vi "ABR3-Channel Assignments.vi"(0 "Stimulus":T5={"Ear"=enum."Left", "Waveform"=enum."TONE PIP", "Frequency (kHz)"="", "Rep rate (/sec)"=30.0, "Alternate Polarity"=FALSE, "WavFiles"="", "Level (dB SPL)"=30.0, "WavFolder"=path "", "Chirp"={"Type"=enum."AN latency-corrected", "Duration (ms)"=0.0, "Fmin (kHz)"=0.0, "Fmax (kHz)"=0.0, "precompensate"=FALSE}, "Noise"={"Seed"=0, "InvFilt"=FALSE, "AWeight"=FALSE, "afile"=path "", "Filter"={"Type"=enum."Lowpass", "CF (kHz)"=0.0, "BW (kHz)"=0.0, "Cascade"=FALSE, "Quadrature"=FALSE, "Scale Factor"=0.0, "Stages"=[], "Class"=enum."Elliptic", "Order"=0, "BWUnits"=enum."Linear"}}}, 1 "Masker":T2, 11 "error in (no error)":errorcluster) -> (15 "error out":errorcluster)   [LabVIEW 2020]
uses:
  TypeDefs/ABR3-Stimulus.ctl
  Utility VIs/Type Defs/Left-Right ring.ctl
  TypeDefs/ABR-Waveform Enum.ctl
  Signal Synthesis VIs/Controls/Advanced Filter XCtl/Advanced Filter XCtl.xctl
  TypeDefs/ABR3-Masker Spec.ctl
  Signal Synthesis VIs/Controls/Level XCtl/Level XCtl.xctl
  Utility VIs/Type Defs/Speaker ring.ctl
panel:
  out "Masker channels":T1[](array[typedef])
  out "Unused secondary channels":T1[](array[typedef])
  out "Signal channels":T1[](array[typedef])
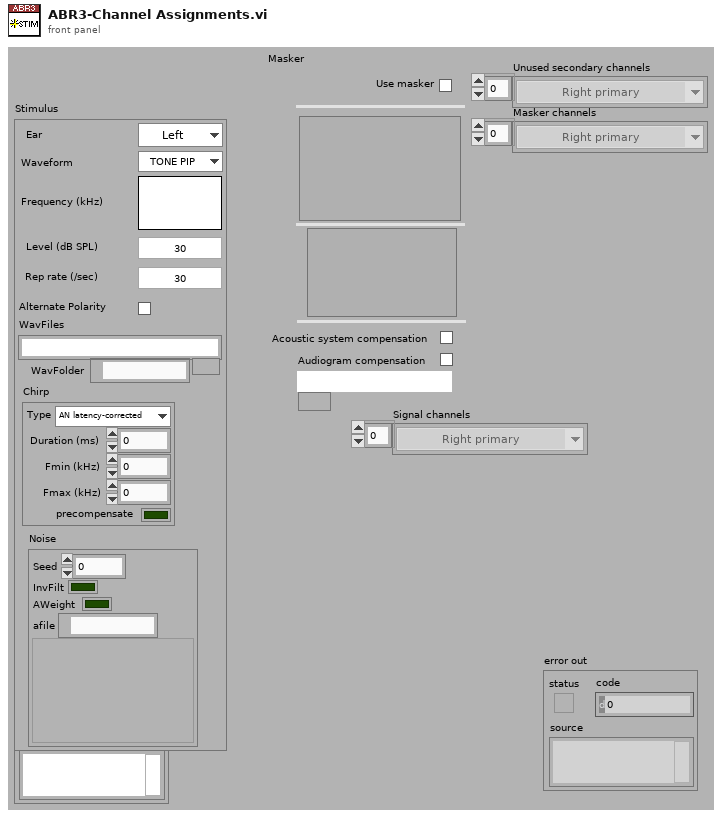
[diagram p1: front panel]
types:
  T1 = typedef "Speaker ring.ctl" = enum16{"Right primary", "Right secondary", "Left primary", "Left secondary"}
  T2 = typedef "ABR3-Masker Spec.ctl" = cluster{"Filter":cluster{"Type":enum16{"Lowpass", "Highpass", "Bandpass", "Bandstop", "OFF"}, "CF (kHz)":dbl, "BW (kHz)":dbl, "Cascade":bool, "Quadrature":bool, "Scale Factor":dbl, "Stages":cluster{"IIR Filter":cluster{"filter structure":enum32{"IIR 2nd Order", "IIR 4th Order"}, "Reverse Coefficients":dbl[], "Forward Coefficients":dbl[]}, "State":dbl[]}[], "Class":enum16{"Elliptic", "Butterworth"}, "Order":i32, "BWUnits":T3}, "Use masker":bool, "Level":cluster{"Level":dbl, "Units":T4, "Max":dbl, "Multiplier":dbl, "Cal File":path, "Cal":cluster{"Freq (Hz)":dbl[], "Mag (dB SPL)":dbl[], "Phase (deg)":dbl[]}}, "Audiogram Comp":bool, "Audiogram File":path, "InvFilt":bool}
  T3 = typedef "Filter-Bandwidth Units.ctl" = enum16{"Linear", "Octaves", "Min-Max"}
  T4 = typedef "Level Units.ctl" = enum16{"dB atten", "dB SPL", "dB re 1 Vrms", "dB V/Hz½", "mW", "dB HL", "Volts", "dB mW"}
  T5 = typedef "ABR3-Stimulus.ctl" = cluster{"Ear":T6, "Waveform":T7, "Frequency (kHz)":string, "Rep rate (/sec)":dbl, "Alternate Polarity":bool, "WavFiles":string, "Level (dB SPL)":dbl, "WavFolder":path, "Chirp":cluster{"Type":enum16{"AN latency-corrected", "Arbitrary"}, "Duration (ms)":dbl, "Fmin (kHz)":dbl, "Fmax (kHz)":dbl, "precompensate":bool}, "Noise":cluster{"Seed":i32, "InvFilt":bool, "AWeight":bool, "afile":path, "Filter":cluster{"Type":enum16{"Lowpass", "Highpass", "Bandpass", "Bandstop", "OFF"}, "CF (kHz)":dbl, "BW (kHz)":dbl, "Cascade":bool, "Quadrature":bool, "Scale Factor":dbl, "Stages":cluster{"IIR Filter":cluster{"filter structure":enum32{"IIR 2nd Order", "IIR 4th Order"}, "Reverse Coefficients":dbl[], "Forward Coefficients":dbl[]}, "State":dbl[]}[], "Class":enum16{"Elliptic", "Butterworth"}, "Order":i32, "BWUnits":T3}}}
  T6 = typedef "Left-Right ring.ctl" = enum16{"Right", "Left"}
  T7 = typedef "ABR-Waveform Enum.ctl" = enum16{"TONE PIP", "CLICK", "FILE", "CHIRP", "NOISE", "VERHULST"}
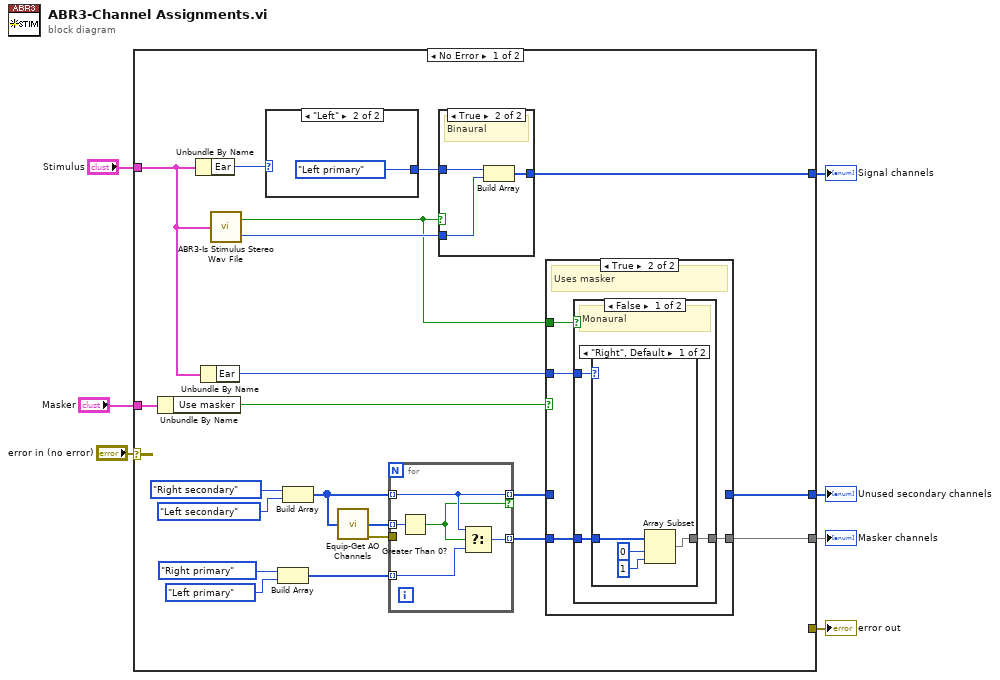
[diagram p0: block diagram]
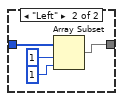
[diagram p3: hidden frame]
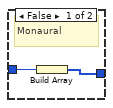
[diagram p5: hidden frame]
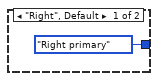
[diagram p6: hidden frame]
diagram:
  n1 = case shown="No Error" "error in (no error)" {
    selector: "error in (no error)" -> [_ w58]
    tunnel: "Stimulus" -> [w14 _]
    tunnel: [_ w58] -> w5
    tunnel: "Masker" -> [w25 _]
    tunnel: [w10 _] -> w3
    tunnel: [w9 _] -> w2
    tunnel: [w8 _] -> w1
    frame No Error {
      n2 = Unbundle By Name(w25) -> ("Use masker"=w16:bool)
      n3 = Unbundle By Name(w14) -> ("Ear"=w28:T6)
      n4 = Unbundle By Name(w14) -> ("Ear"=w13:T6)
      n5 = call "ABR3-Is Stimulus Stereo Wav File.vi"("Stimulus"=w14) -> ("Is Stereo Wav File"=w12:bool, "Channel To Add"=w27:T1)
      n6 = case shown="\"Left\"" w28 {
        tunnel: [Speaker_ring."Right primary" ("Speaker") Speaker_ring."Left primary" ("Speaker")] -> w26
        frame "Right", Default {
        }
        frame "Left" {
        }
      }
      n7 = Build Array(Speaker_ring."Right primary" ("Speaker"), Speaker_ring."Left primary" ("Speaker")) -> (w19:T1[])
      n8 = Build Array(Speaker_ring."Right secondary" ("Speaker"), Speaker_ring."Left secondary" ("Speaker")) -> (w17:T1[])
      n9 = call "Equip-Get AO Channels.vi"("Outputs"=w17) -> ("AO Channels"=w18:i32[], "error out"=w20:errorcluster)  [unwired: 13 in]
      n10 = for {
        tunnel: w18 -> [w50] mode=indexing
        tunnel: w20 -> [_]
        tunnel: w19 -> [w49] mode=indexing
        tunnel: [w48] -> w15 mode=indexing
        tunnel: w17 -> [w47] mode=indexing
        tunnel: [w47] -> w11 mode=indexing if=w46
        n11 = Greater Than 0?(x=w50) -> (x > 0?=w46:bool)
        n12 = Select(t=w47, s=w46, f=w49) -> (s? t:f=w48:T1)
      }
      n13 = case shown="True" w12 {
        tunnel: w27 -> [_ w54]
        tunnel: w26 -> [w52 w55]
        tunnel: [w51 w53] -> w10
        frame False {
          # "Monaural"
          n14 = Build Array(w52) -> (w51:T1[])
        }
        frame True {
          # "Binaural"
          n15 = Build Array(w55, w54) -> (w53:T1[])
        }
      }
      n16 = case shown="True" w16 {
        tunnel: w15 -> [_ w32]
        tunnel: w13 -> [_ w30]
        tunnel: w12 -> [_ w33]
        tunnel: w11 -> [w29 _]
        tunnel: [_ w31] -> w8
        tunnel: [w29 _] -> w9
        frame False {
        }
        frame True {
          # "Uses masker"
          n17 = case shown="False" w33 {
            tunnel: w32 -> [w36 w45]
            tunnel: [w34 w45] -> w31
            tunnel: w30 -> [w35 _]
            frame False {
              # "Monaural"
              n18 = case shown="\"Right\", Default" w35 {
                tunnel: w36 -> [w38 w44]
                tunnel: [w37 w41] -> w34
                frame "Right", Default {
                  n19 = Array Subset(array=w38, index=0, length=1) -> (w37:T1[])
                }
                frame "Left" {
                  n20 = Array Subset(array=w44, index=1, length=1) -> (w41:T1[])
                }
              }
            }
            frame True {
              # "Binaural"
            }
          }
        }
      }
    }
    frame Error {
    }
  }
  "error out" <- w5
  "Signal channels" <- w3
  "Unused secondary channels" <- w2
  "Masker channels" <- w1
